vi "FMDemod (SubVI).vi"(10 "Cluster":cluster{"Interpolation":i32, "Decimation":i32}, 11 "buf in":u8[](array[numeric])) -> (0 "Waveform":waveform(dbl), 1 "Complex Wave":cdb[](array[numeric]))   [LabVIEW 2013]
uses:
  <vilib>/Analysis/3filter.llb/Filter Passband Type.ctl
  <vilib>/Analysis/3filter.llb/Butterworth Filter (CDB).vi
  <vilib>/Analysis/3filter.llb/FIR Filter (DBL).vi
  <vilib>/Analysis/2dsp.llb/Rational Resample (single channel, DBL).vi
  <vilib>/Analysis/2dsp.llb/Decimate (continuous, CDB).vi
  <vilib>/Analysis/NI_AALPro.lvlib
  <vilib>/Analysis/NI_AALBase.lvlib
panel:
  out "XY Graph":cdb[](graph)
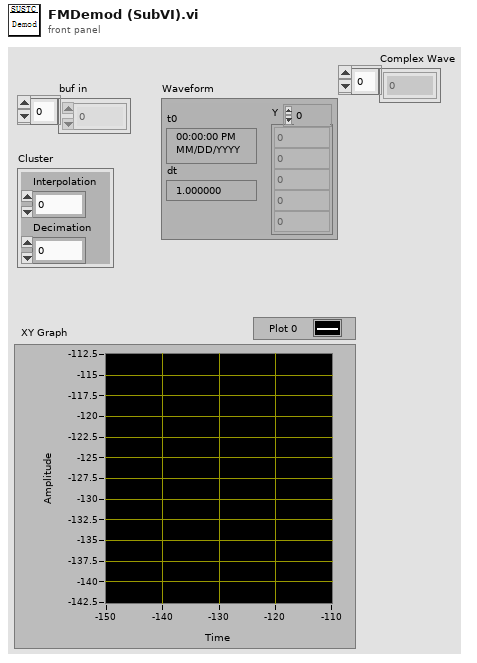
[diagram p1: front panel]
types:
  T1 = typedef "NI_AALBase.lvlib/Filter Passband Type.ctl" = enum32{"Lowpass", "Highpass", "Bandpass", "Bandstop"}
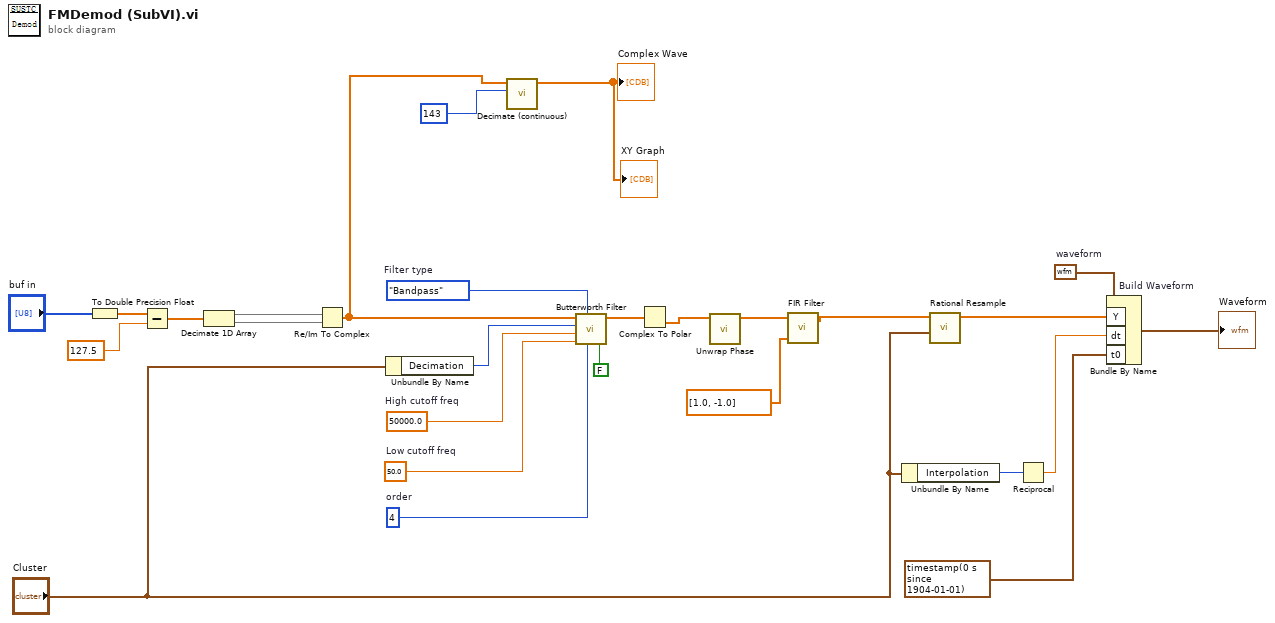
[diagram p0: block diagram]
diagram:
  w5 = waveform(dbl) {"t0"=timestamp(0 s since 1904-01-01), "dt"=1.0, "Y"=[]}  # waveform
  w10 = 50.0  # Low cutoff freq
  w13 = 4  # order
  w12 = Filter_Passband_Type."Bandpass"  # Filter type
  w11 = 50000.0  # High cutoff freq
  n1 = To Double Precision Float(number="buf in") -> (double precision float=w16:dbl[])
  n2 = Subtract(x=w16, y=127.5) -> (x-y=w18:dbl[])
  n3 = Decimate 1D Array "Decimate 1D Array"(w18) -> (w20:dbl[], w19:dbl[])
  n4 = Re/Im To Complex(1:w19, 2:w20) -> (0:w2:cdb[])
  n5 = Unbundle By Name("Cluster") -> ("Decimation"=w6:i32)
  n6 = call-poly <vilib>:"Decimate (continuous).vi"("decimating factor"=143, "X"=w2) -> ("Decimated Array"=→"Complex Wave" →"XY Graph":cdb[])  [unwired: 8 in, 1 out]
  n7 = call-poly <vilib>:"Butterworth Filter.vi"("init/cont (init:F)"=FALSE, "order"=w13, "filter type"=w12, "low cutoff freq: fl"=w10, "high cutoff freq: fh"=w11, "sampling freq: fs"=w6, "X"=w2) -> ("Filtered X"=w8:cdb[])  [unwired: 1 in, 1 out]
  n8 = Complex To Polar(r * e^(i*theta)=w8) -> (theta=w4:dbl[])  [unwired: 1 out]
  n9 = call <vilib>:"Unwrap Phase.vi"("Phase"=w4) -> ("Unwrapped Phase"=w23:dbl[])  [unwired: 9 in, 1 out]
  n10 = call-poly <vilib>:"FIR Filter.vi"("FIR Coefficients"=dbl[] [1.0, -1.0], "X"=w23) -> ("Filtered X"=w24:dbl[])  [unwired: 2 in, 1 out]
  n11 = Unbundle By Name("Cluster") -> ("Interpolation"=w26:i32)
  n12 = call-poly <vilib>:"Rational Resample.vi"("resample factor"="Cluster", "X"=w24) -> ("Y"=w15:dbl[])  [unwired: 7 in, 2 out]
  n13 = Reciprocal(x=w26) -> (1/x=w27:dbl)
  n14 = Bundle By Name "Build Waveform"(cluster=w5, "Y"=w15, "dt"=w27, "t0"=timestamp(0 s since 1904-01-01)) -> (→"Waveform":waveform(dbl))
